vi "CRYSet Messages Run Front Panel.vi"(11 "Vi Ref":refnum<vi>) -> ()   [LabVIEW 2013]
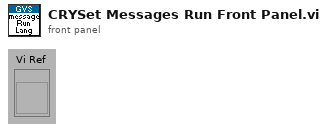
[diagram p1: front panel]
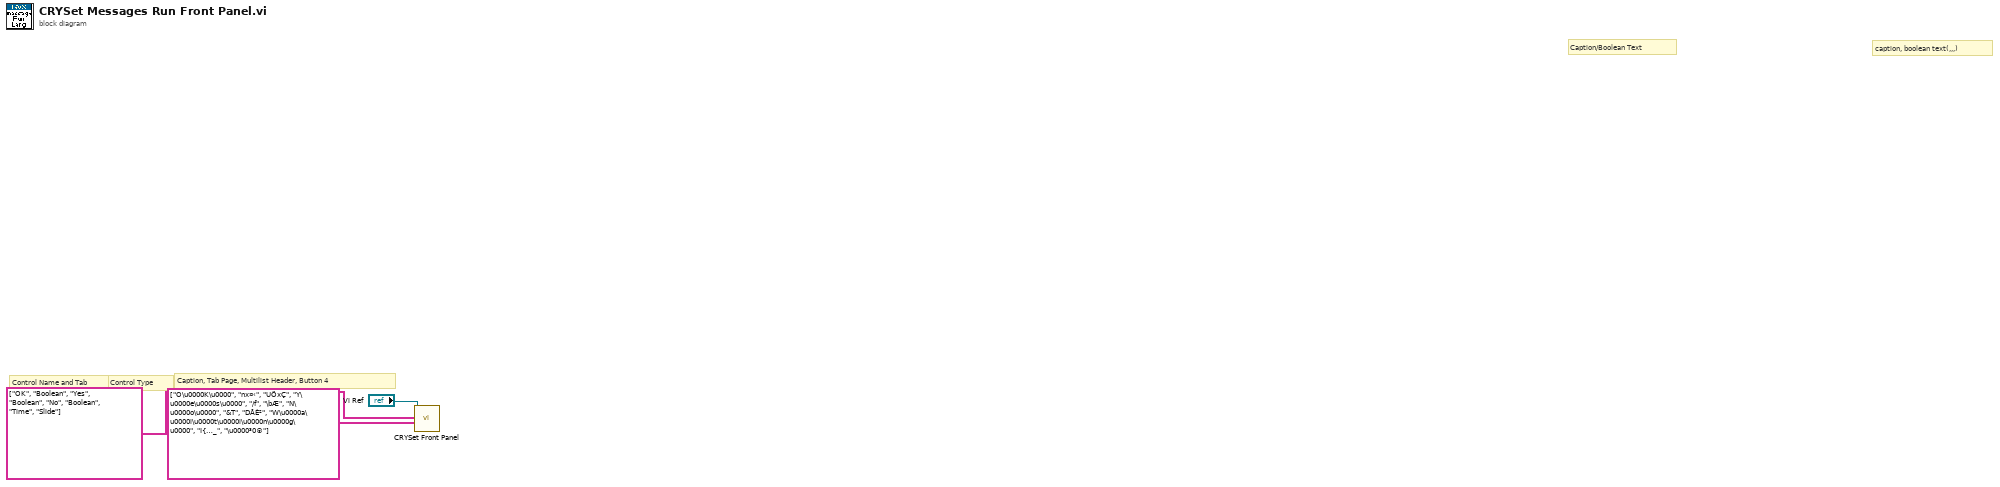
[diagram p0: block diagram]
diagram:
  # "Caption, Tab Page, Multilist Header, Button 4"
  # "Control Type"
  # "Control Name and Tab"
  # "caption, boolean text(,,,)"
  # "Caption/Boolean Text"
  n1 = call "CRYSet Front Panel.vi"("Caption(Boolean Text)"=string[][] [["O\u0000K\u0000", "nx¤‹", "UÖxÇ"], ["Y\u0000e\u0000s\u0000", "/f", "\bÆ"], ["N\u0000o\u0000", "&T", "DÅÈ²"], ["W\u0000a\u0000i\u0000t\u0000i\u0000n\u0000g\u0000", "I{…_", "\u0000³0®"]], "Control ID and Type(Label Name, Type)"=string[][] [["OK", "Boolean"], ["Yes", "Boolean"], ["No", "Boolean"], ["Time", "Slide"]], "Vi Ref"="Vi Ref") -> ()  [unwired: 9 in]
